vi "sub_udp_master-senddata.vi"(11 "index":i32) -> (3 "udp send data":string)   [LabVIEW 2019]
uses:
  Ctrl/gps-databuf.ctl
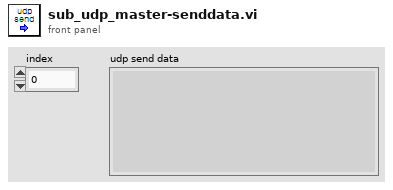
[diagram p1: front panel]
types:
  T1 = typedef "gps-databuf.ctl" = enum16{"read", "write"}
  T2 = cluster{"System Feedback":cluster{"system state":string, "Control Mode":u8, "Battery Voltage":dbl, "error code High":u8, "error code Low":u8}, "Motion Feedback":cluster{"Linear Velocity (m/s)":dbl, "Angular Velocity (rad/s)":dbl}}
  T3 = cluster{"rawdata":string, "GPS Data":cluster{"Latitude":cluster{"Valid?":bool, "Latitude (Deg)":dbl}, "Longitude":cluster{"Valid?":bool, "Longitude (Deg)":dbl}, "Height":cluster{"Valid?":bool, "Height (m)":dbl}, "Undulation":cluster{"Valid?":bool, "Undulation(m)":dbl}, "North Vel":cluster{"Valid?":bool, "North Vel (m/s)":dbl}, "East Vel":cluster{"Valid?":bool, "East Vel (m/s)":dbl}, "Up Vel":cluster{"Valid?":bool, "Up Vel (m/s)":dbl}, "Roll":cluster{"Valid?":bool, "Roll (degrees)":dbl}, "Pitch":cluster{"Valid?":bool, "Pitch (degrees)":dbl}, "Azimuth":cluster{"Valid?":bool, "Azimuth (degrees)":dbl}, "Lat deviation":cluster{"Valid?":bool, "Lat deviation (m)":dbl}, "Long deviation":cluster{"Valid?":bool, "Long deviation (m)":dbl}, "Height deviation":cluster{"Valid?":bool, "Height deviation (m)":dbl}, "North vel deviation":cluster{"Valid?":bool, "North vel deviation (m/s)":dbl}, "East vel deviation":cluster{"Valid?":bool, "East vel deviation (m/s)":dbl}, "Up vel deviation":cluster{"Valid?":bool, "Up vel deviation (m/s)":dbl}, "Roll deviation":cluster{"Valid?":bool, "Roll deviation (degrees)":dbl}, "Pitch deviation":cluster{"Valid?":bool, "Pitch deviation (degrees)":dbl}, "Azimuth deviation":cluster{"Valid?":bool, "Azimuth deviation (degrees)":dbl}, "Ext sol status":cluster{"Valid?":bool, "Ext sol status":dbl}}, "Heading":dbl, "utm-1":cluster{"XN":dbl, "YE":dbl}}
  T4 = typedef "error_check.ctl" = cluster{"AGV":T5, "AGV Estop":T5, "Obstacle":T5, "GNSS":T5, "TIM571":T5, "Cam":T5, "Joystick":T5}
  T5 = typedef "status.ctl" = u16
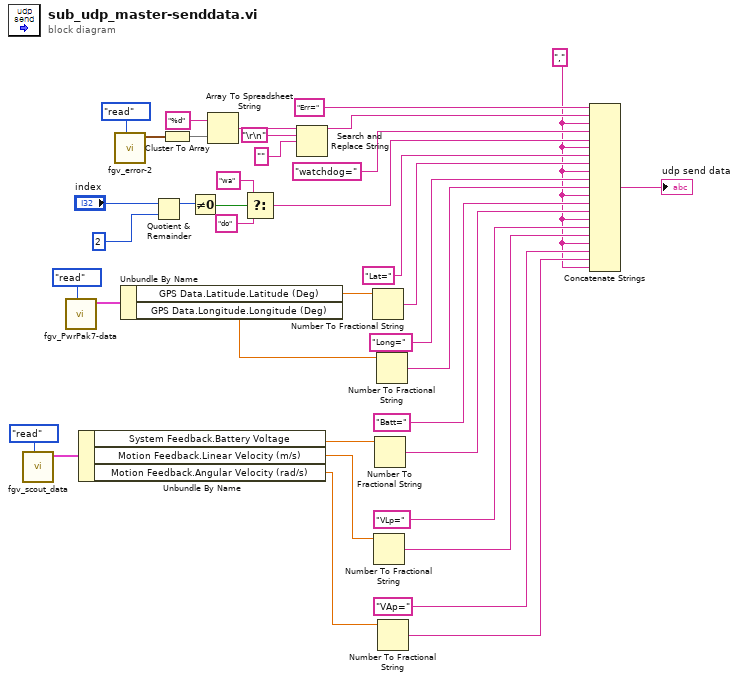
[diagram p0: block diagram]
diagram:
  w1 = "," ("문자열")
  n1 = call "fgv_scout_data.vi"("cmd"=enum16{"write", "read"}."read") -> ("agv data out"=w10:T2)  [unwired: 9 in, 1 out]
  n2 = call "fgv_PwrPak7-data.vi"("cmd"=gps-databuf."read") -> ("data cluster out"=w19:T3)  [unwired: 9 in, 1 out]
  n3 = Unbundle By Name(w10) -> ("System Feedback.Battery Voltage"=w9:dbl, "Motion Feedback.Linear Velocity (m/s)"=w7:dbl, "Motion Feedback.Angular Velocity (rad/s)"=w6:dbl)
  n4 = call "fgv_error-2.vi"("cmd"=enum16{"init", "read", "write"}."read") -> ("Error Display"=w22:T4)  [unwired: 9 in, 1 out]
  n5 = Unbundle By Name(w19) -> ("GPS Data.Latitude.Latitude (Deg)"=w18:dbl, "GPS Data.Longitude.Longitude (Deg)"=w17:dbl)
  n6 = Quotient & Remainder(x="index", y=2) -> (x-y*floor(x/y)=w34:i32)  [unwired: 1 out]
  n7 = Cluster To Array(cluster=w22) -> (array=w23:T5[])
  n8 = Not Equal To 0?(x=w34) -> (x != 0?=w35:bool)
  n9 = Array To Spreadsheet String(array=w23, 3:"%d" ("포맷 문자열")) -> (spreadsheet string=w25:string)  [unwired: 1 in]
  n10 = Select(t="wa" ("포맷 문자열"), s=w35, f="do" ("포맷 문자열")) -> (s? t:f=w38:string)
  n11 = Search and Replace String(input string=w25, search string="\r\n", replace string="" ("대체 문자열(\"\")")) -> (result string=w29:string)  [unwired: 5 in, 3 out]
  n12 = Number To Fractional String(number=w18) -> (F-format string=w15:string)  [unwired: 3 in]
  n13 = Number To Fractional String(number=w7) -> (F-format string=w4:string)  [unwired: 3 in]
  n14 = Number To Fractional String(number=w9) -> (F-format string=w8:string)  [unwired: 3 in]
  n15 = Number To Fractional String(number=w17) -> (F-format string=w13:string)  [unwired: 3 in]
  n16 = Number To Fractional String(number=w6) -> (F-format string=w2:string)  [unwired: 3 in]
  n17 = Concatenate Strings("Err=" ("문자열"), w29, w1, "watchdog=" ("문자열"), w38, w1, "Lat=" ("문자열"), w15, w1, "Long=" ("문자열"), w13, w1, "Batt=" ("문자열"), w8, w1, "VLp=" ("문자열"), w4, w1, "VAp=" ("문자열"), w2, w1) -> (→"udp send data":string)
